vi "Get Fit Parameter Names, Values & Uncertainties.vi"(8 "error in (no error)":errorcluster, 9 "Fit Parameter Uncertainties":variant, 11 "Fit Parameters":variant) -> (0 "Error Out":errorcluster, 1 "Fit Parameter Uncertainties":dbl[](array[numeric]), 2 "Fit Parameter Values":dbl[](array[numeric]), 3 "Fit Parameter Names":string[](array[string]))   [LabVIEW 2019]
uses:
  Variant to Data.lvlib
  Variant to Boolean.vi
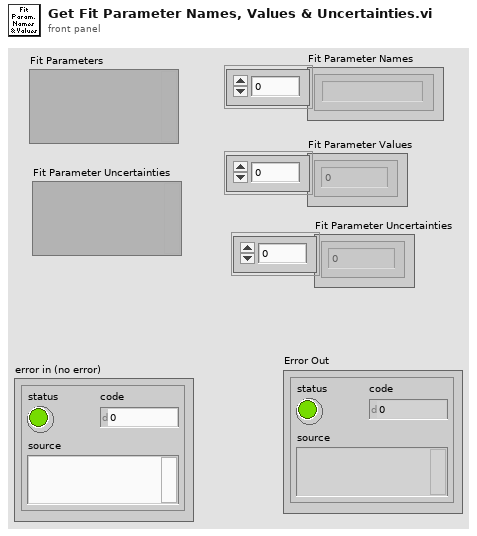
[diagram p1: front panel]
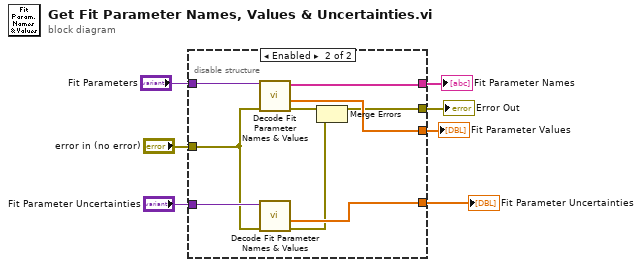
[diagram p0: block diagram]
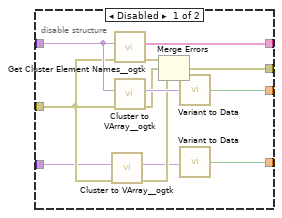
[diagram p2: hidden frame]
diagram:
  n1 = disable-structure shown="Enabled" {
    disable-tunnel: [w19 w24] -> w7
    disable-tunnel: [w17 w25] -> w6
    disable-tunnel: "Fit Parameters" -> [w16 w27]
    disable-tunnel: [w14 w20] -> w4
    disable-tunnel: "error in (no error)" -> [w12 w26]
    disable-tunnel: [w11 w23] -> w2
    disable-tunnel: "Fit Parameter Uncertainties" -> [w9 w28]
    frame Disabled {
      n2 = call <userlib>:"Cluster to VArray__ogtk.vi"("error in (no error)"=w12, "Cluster"=w9) -> ("error out"=w10:errorcluster, "VArray"=w8:variant)  [unwired: 8 in]
      n3 = call <userlib>:"Get Cluster Element Names__ogtk.vi"("error in (no error)"=w12, "Cluster"=w16) -> ("error out"=w13:errorcluster, "Element Names"=w17:string[])  [unwired: 8 in]
      n4 = call <userlib>:"Cluster to VArray__ogtk.vi"("error in (no error)"=w12, "Cluster"=w16) -> ("error out"=w15:errorcluster, "VArray"=w18:variant)  [unwired: 8 in]
      n5 = Merge Errors(w13, w15, w10) -> (w14:errorcluster)
      n6 = call-poly "Variant to Data.vi"("Variant"=w18) -> ("Value"=w19:bool)  [unwired: 8 in]
      n7 = call-poly "Variant to Data.vi"("Variant"=w8) -> ("Value"=w11:bool)  [unwired: 8 in]
    }
    frame Enabled {
      n8 = call "Decode Fit Parameter Names & Values.vi"("Error In"=w26, "Fit Parameters"=w27) -> ("Error Out"=w22:errorcluster, "Parameter Values"=w24:dbl[], "Parameter Names"=w25:string[])  [unwired: 7 in]
      n9 = call "Decode Fit Parameter Names & Values.vi"("Error In"=w26, "Fit Parameters"=w28) -> ("Error Out"=w21:errorcluster, "Parameter Values"=w23:dbl[])  [unwired: 7 in, 1 out]
      n10 = Merge Errors(w22, w21) -> (w20:errorcluster)
    }
  }
  "Fit Parameter Values" <- w7
  "Fit Parameter Names" <- w6
  "Error Out" <- w4
  "Fit Parameter Uncertainties" <- w2
